vi "Get All FTC Data.vi"(11 "NXT":T1) -> (0 "Teleop?":bool, 1 "Stopped?":bool, 2 "Enabled?":enum16{"Disabled", "Enabled"}(ring), 3 "NXT":T1, 4 "Packet Received?":bool, 5 "Controller 2":string, 6 "Online?":bool, 7 "Controller 1":string)   [LabVIEW 2012, in "FTC.lvlib"]
uses:
  FTC.lvlib
  <vilib>/NXT/Subs/LVHSConnector.ctl
  <vilib>/NXT/LegoClasses/BrickReference/BrickReference.lvclass
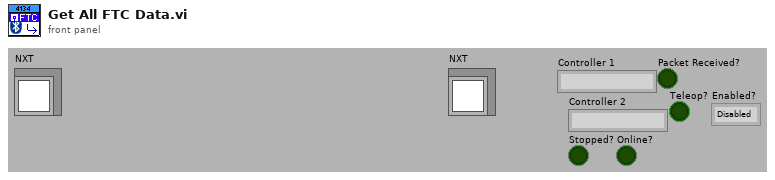
[diagram p1: front panel]
types:
  T1 = typedef "LVHSConnector.ctl" = refnum<class "BrickReference.lvclass">
  T2 = cluster{"Controller 1":string, "Controller 2":string, "Stopped?":bool, "Online?":bool, "Packet Received?":bool, "Teleop?":bool, "Enabled?":enum16{"Disabled", "Enabled"}}
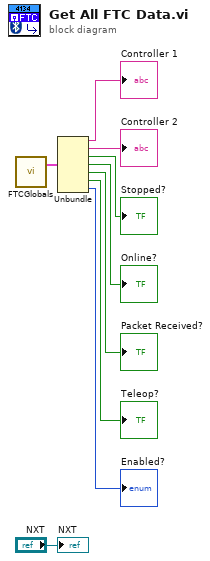
[diagram p0: block diagram]
diagram:
  n1 = call "FTCGlobals.vi"() -> ("Read Globals"=w8:T2)  [unwired: 4 in]
  n2 = Unbundle(w8) -> ("Controller 1"=→"Controller 1":string, "Controller 2"=→"Controller 2":string, "Stopped?"=→"Stopped?":bool, "Online?"=→"Online?":bool, "Packet Received?"=→"Packet Received?":bool, "Teleop?"=→"Teleop?":bool, "Enabled?"=→"Enabled?":enum16{"Disabled", "Enabled"})
  "NXT" <- "NXT"
